vi "数据处理.vi"(6 "电阻值":dbl, 7 "数据显示输入":string[][](array[string]), 9 "列数":i32, 10 "行数":i32, 11 "数据显示":refnum<vi>) -> (5 "数据显示输出":string[][](array[string]))   [LabVIEW 2015]
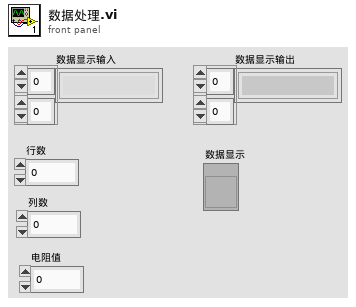
[diagram p1: front panel]
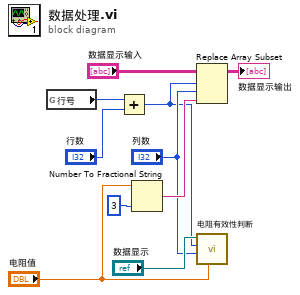
[diagram p0: block diagram]
diagram:
  n1 = global read "全局.vi" "行号"() -> (w3:i32)
  n2 = Add(x=w3, y="行数") -> (x+y=w1:i32)
  n3 = Number To Fractional String(number="电阻值", precision (6)=i16 3 ("精度(6)")) -> (F-format string=w9:string)  [unwired: 2 in]
  n4 = Replace Array Subset(array="数据显示输入", new element=w9, index (row)=w1, index (col)="列数") -> (→"数据显示输出":string[][])
  n5 = call "电阻有效性判断.vi"("温度值"="电阻值", "Column"="列数", "行数"=w1, "Table输入"="数据显示") -> ()  [unwired: 8 in]
